vi "ArbitraryPosition.vi"() -> ()   [LabVIEW 2014]
panel:
  in  "Y":dbl
  in  "Z":dbl
  in  "X":dbl
  out "pfVoltage Z":sgl
  out "pfVoltage Y":sgl
  out "pfVoltage X":sgl
  out "error out":errorcluster
  in  "MG17Piezo X":refnum<k7>(container)
  in  "MG17Piezo Y":refnum<k7>(container)
  in  "MG17Piezo Z":refnum<k7>(container)
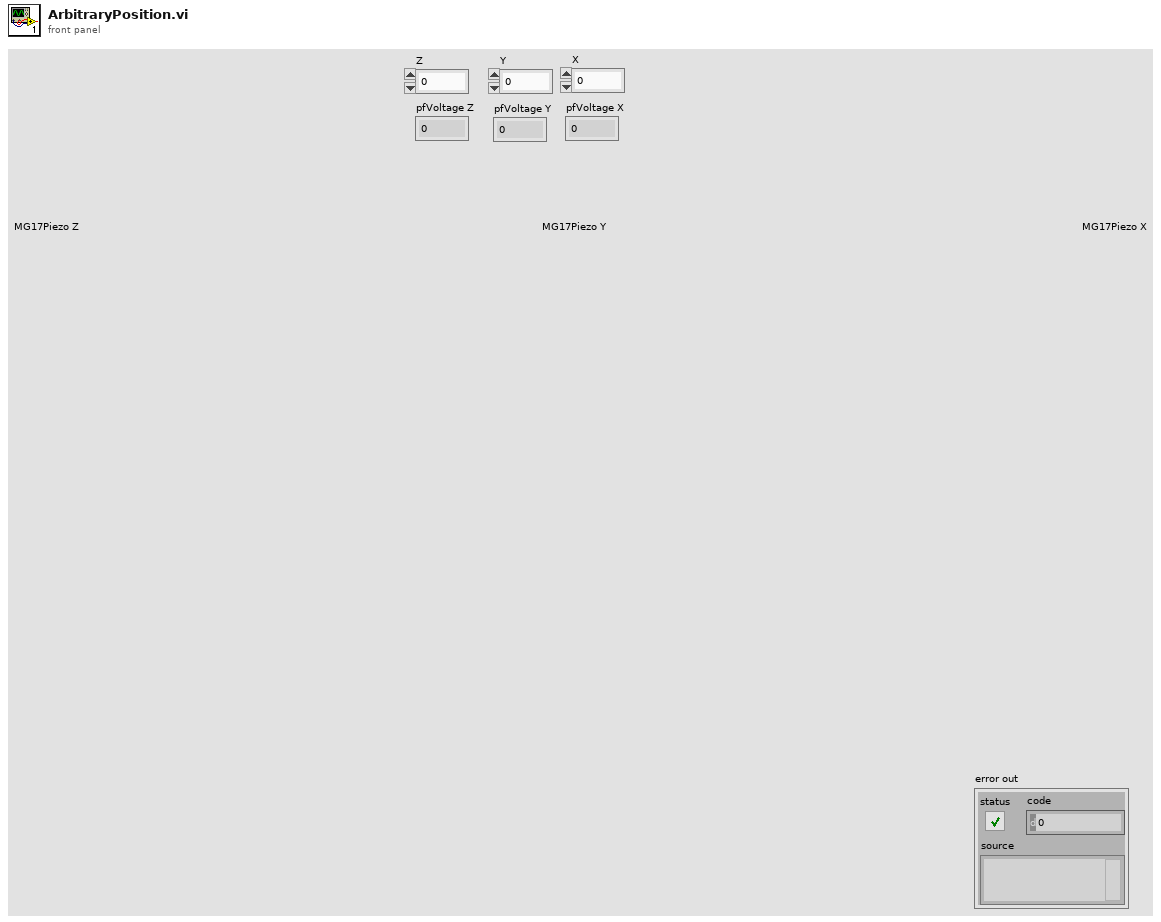
[diagram p1: front panel]
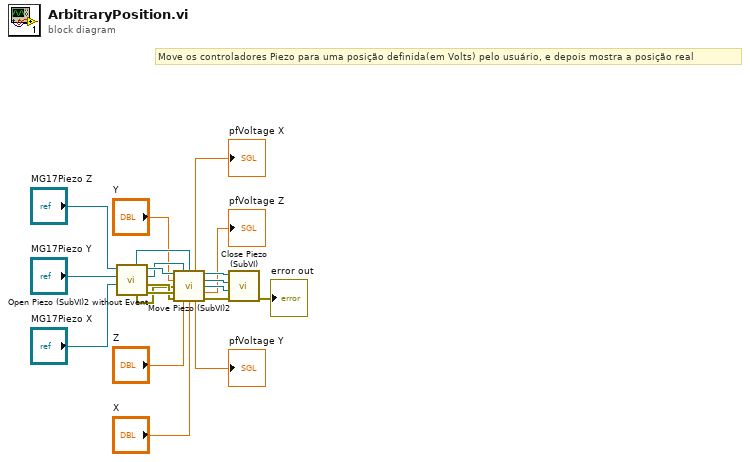
[diagram p0: block diagram]
diagram:
  # "Move os controladores Piezo para uma posição definida(em Volts) pelo usuário, e depois mostra a posição real"
  n1 = call "Open Piezo (SubVI)2 without Event.vi"("MG17Piezo X"="MG17Piezo X", "MG17Piezo Y"="MG17Piezo Y", "MG17Piezo Z"="MG17Piezo Z") -> ("error out Z"=w13:errorcluster, "error out Y"=w12:errorcluster, "MG17 X"=w14:refnum<k7>, "MG17 Y"=w15:refnum<k7>, "error out X"=w11:errorcluster, "MG17 Z"=w16:refnum<k7>)  [unwired: 3 in]
  n2 = call "Move Piezo (SubVI)2.vi"("MG17 Y in"=w15, "MG17 X in"=w14, "MG17 Z in"=w16, "Y"="Y", "error in X"=w11, "error in Z"=w13, "error in Y"=w12, "Z"="Z", "X"="X") -> ("pfVoltage X"=→"pfVoltage X":sgl, "MG17 Y out"=w7:refnum<k7>, "MG17 Z out"=w8:refnum<k7>, "MG17 X out"=w9:refnum<k7>, "pfVoltage Z"=→"pfVoltage Z":sgl, "pfVoltage Y"=→"pfVoltage Y":sgl, "error out"=w10:errorcluster)
  n3 = call "Close Piezo (SubVI).vi"("error in (no error)"=w10, "MG17 X"=w9, "MG17 Z"=w8, "MG17 Y"=w7) -> ("error out"=→"error out":errorcluster)  [unwired: 7 in]
